vi "MasterSlaveDAQ-SplitMaster.vi"() -> ()   [LabVIEW 2014]
doc: "Use this template to build a user interface event handler design pattern. Use this pattern for dialog boxes and other user interfaces. You also can create and execute user-defined events that the VI can handle the same way as user interface events."
uses:
  subVIs/MasterState.ctl
  subVIs/SlaveStateData.ctl
  subVIs/SlaveState.ctl
  <vilib>/Utility/error.llb/DialogType.ctl
  <vilib>/DAQmx/create/channels.llb/DAQmx Create Channel (AI-Voltage-Basic).vi
  <vilib>/DAQmx/configure/timing.llb/DAQmx Timing (Sample Clock).vi
panel:
  in  "File Path":path
  in  "Acquire Data":bool
  in  "Log Data":bool
  in  "File Comment":string
  in  "DAQ Parameters":T1={"physical channels"="", "maximum value"=5.0, "minimum value"=-5.0, "rate"=1000.0, "read period"=0.5} {"read period" format="%0.2f"; "rate" format="%0.2f"; "minimum value" format="%0.2f"; "maximum value" format="%0.2f"}
  in  "quit":bool
  # "V"
  # "V"
  # "Hz"
  # "s"
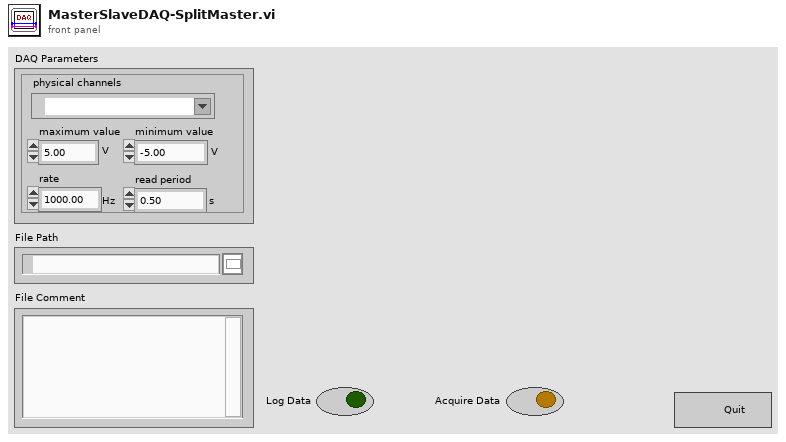
[diagram p1: front panel]
types:
  T1 = cluster{"physical channels":tag, "maximum value":dbl, "minimum value":dbl, "rate":dbl, "read period":dbl}
  T2 = typedef "SlaveStateData.ctl" = cluster{"New State":T3, "DAQ Ref":refnum<k21>, "File Ref":refnum<file>}
  T3 = typedef "SlaveState.ctl" = enum16{"Init", "Idle", "CheckError", "Finalize", "StartDAQ", "AcquireAndLog", "StopDAQ", "UpdateFile"}
  T4 = typedef "MasterState.ctl" = enum16{"Init", "Idle", "CheckError", "Finalize", "ConfigDAQ", "StartDAQ", "AcquireAndLog", "StopDAQ", "ClearDAQ", "OpenFile", "CloseFile"}
  T5 = typedef "DialogType.ctl" = u16
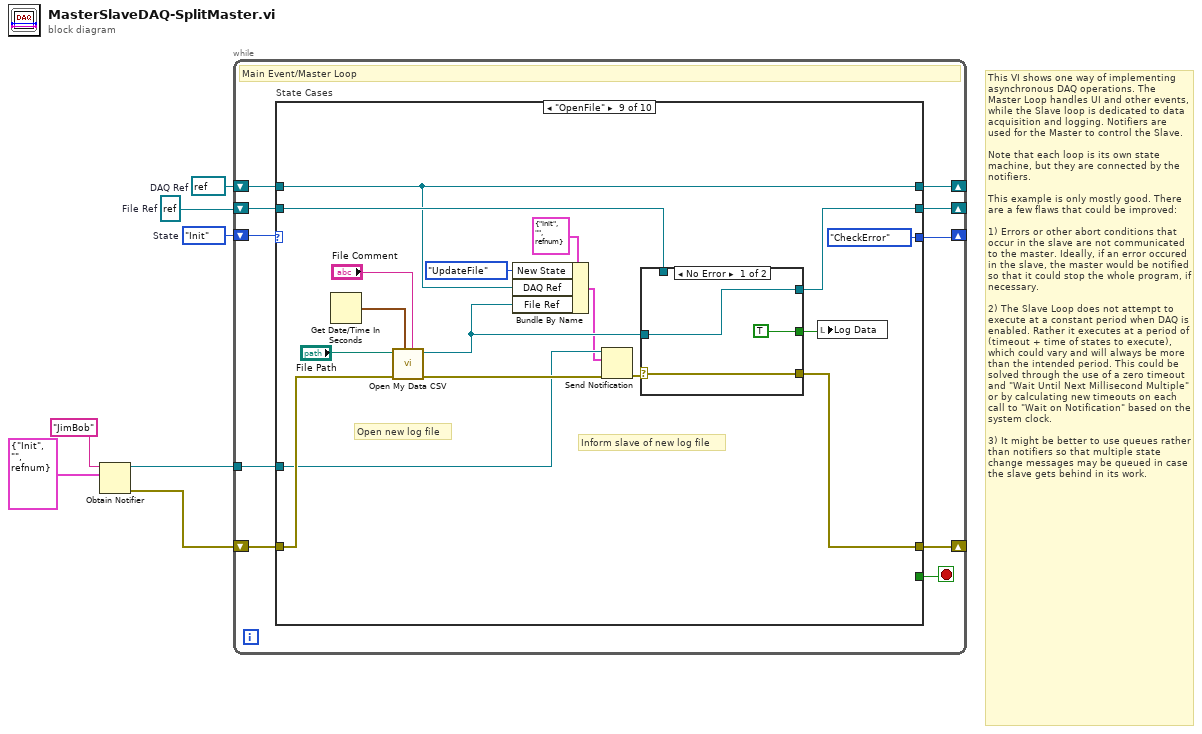
[diagram p0: block diagram]
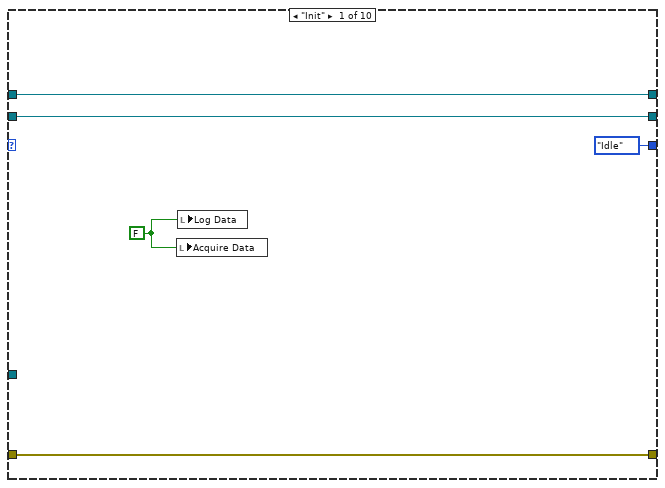
[diagram p2: hidden frame]
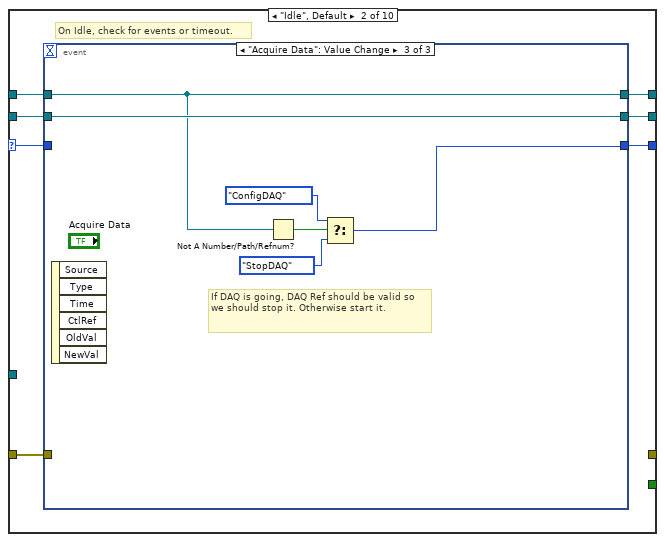
[diagram p3: hidden frame]
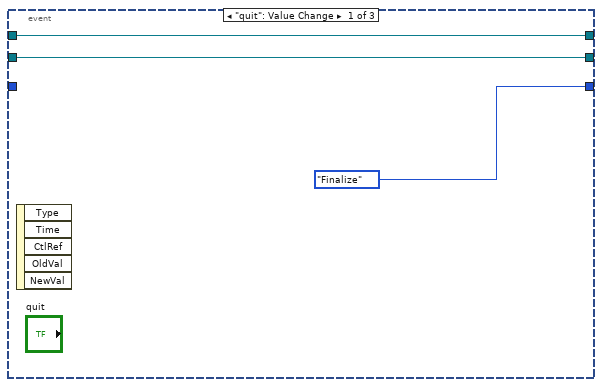
[diagram p4: hidden frame]
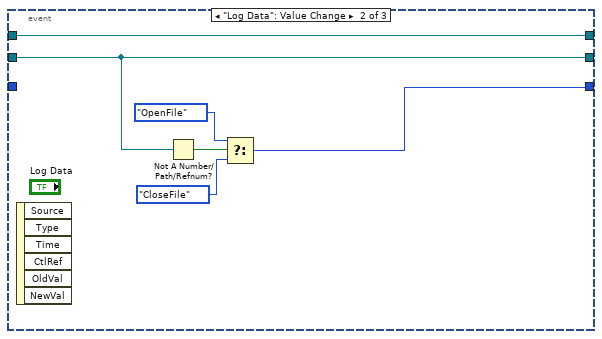
[diagram p5: hidden frame]
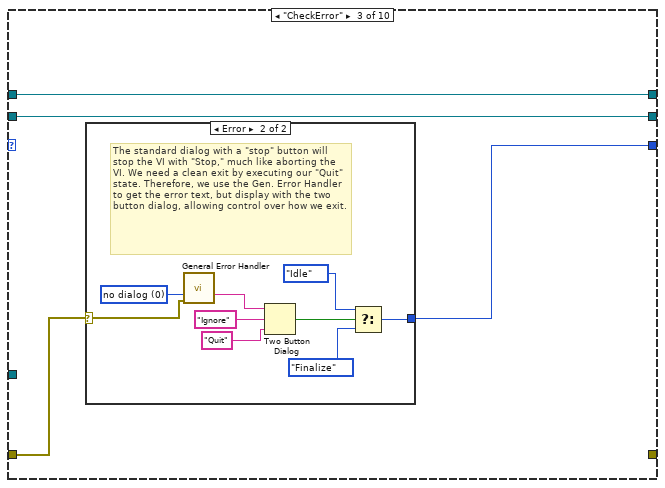
[diagram p6: hidden frame]
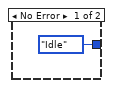
[diagram p7: hidden frame]
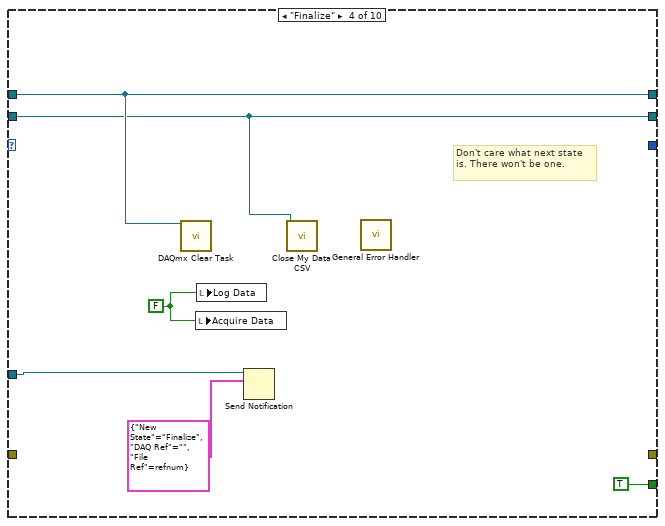
[diagram p8: hidden frame]
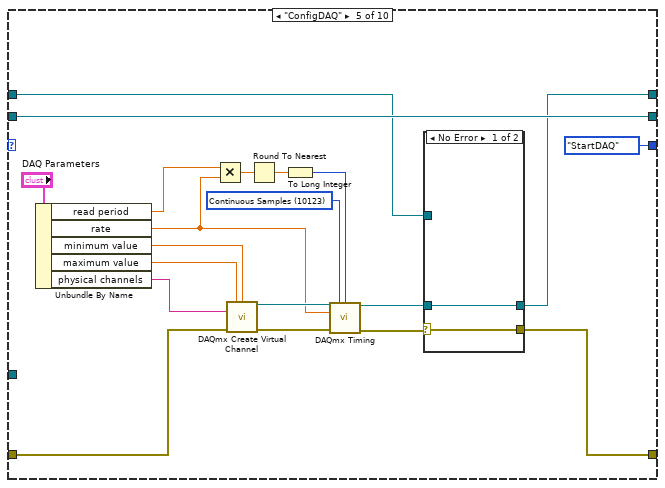
[diagram p9: hidden frame]
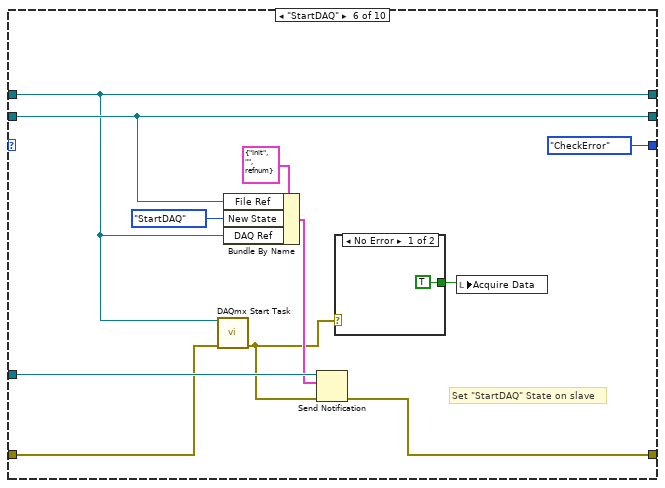
[diagram p11: hidden frame]
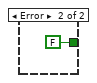
[diagram p12: hidden frame]
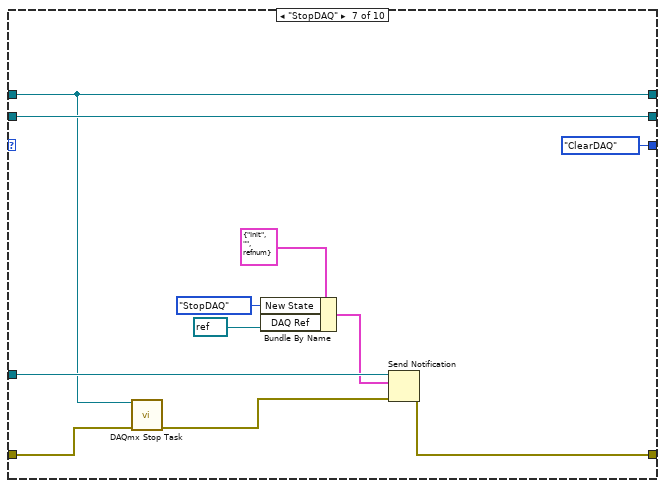
[diagram p13: hidden frame]
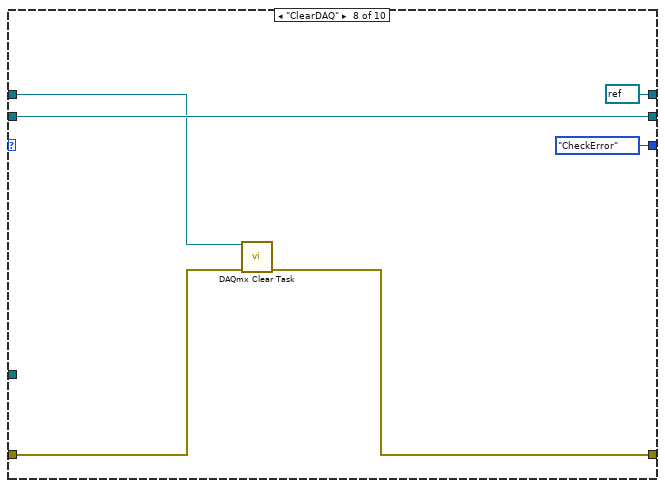
[diagram p14: hidden frame]
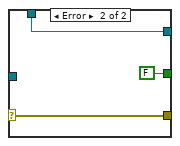
[diagram p15: hidden frame]
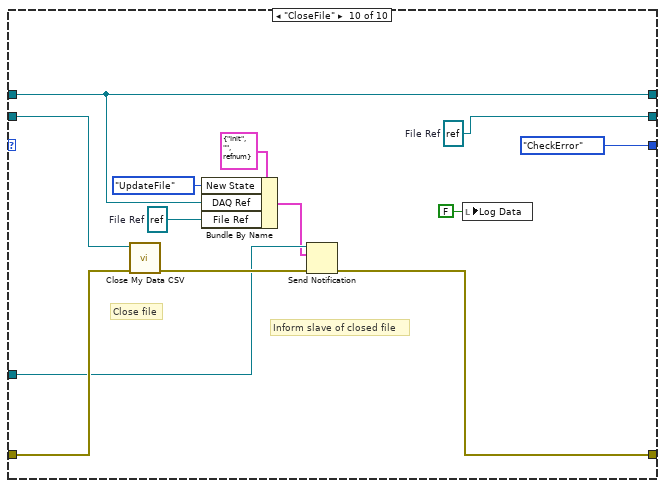
[diagram p16: hidden frame]
diagram:
  w5 = refnum<file> refnum  # File Ref
  w6 = refnum<k21> refnum  # DAQ Ref
  w7 = MasterState."Init"  # State
  # "This VI shows one way of implementing asynchronous DAQ operations. The Master Loop handles UI and other events, while the Slave loop is dedicated to data acquisition and logging. Notifiers are used for the Master to control the Slave.\n\nNote that each loop is its own state machine, but they are connected by the notifiers.\n\nThis example is only mostly good. There are a few flaws that could be improved:\n\n1) Errors or other abort conditions that occur in the slave are not communicated to the master. Ideally, if an error occured in the slave, the master would be notified so that it could stop the whole program, if necessary.\n\n2) The Slave Loop does not attempt to execute at a constant period when DAQ is enabled. Rather it executes at a period of (timeout + time of states to execute), which could vary and will always be more than the intended period. This could be solved through the use of a zero timeout and \"Wait Until Next Millisecond Multiple\" or by calculating new timeouts on each call to \"Wait on Notification\" based on the system clock.\n\n3) It might be better to use queues rather than notifiers so that multiple state change messages may be queued in case the slave gets behind in its work."
  n1 = Obtain Notifier(name (unnamed)="JimBob", notification data type=T2 {"New State"=enum."Init", "DAQ Ref"="", "File Ref"=refnum}) -> (notifier out=w4:refnum<notifier>, error out=w2:errorcluster)  [unwired: 2 in, 1 out]
  n2 = while {
    shift-right: [w16] -> _
    shift-left: w7 -> [w17]
    shift-right: [w15] -> _
    shift-left: w6 -> [w14]
    shift-right: [w13] -> _
    shift-left: w5 -> [w12]
    shift-right: [w11] -> _
    shift-left: w2 -> [w10]
    tunnel: w4 -> [w8]
    stop <- w9 stop-if-true
    # "Main Event/Master Loop"
    n3 = case "State Cases" shown="\"OpenFile\"" w17 {
      selector: w17 -> [_ w29 _ _ _ _ _ _ _ _]
      tunnel: [MasterState."Idle" ("State") w28 w46 _ MasterState."StartDAQ" ("State") MasterState."CheckError" ("State") MasterState."ClearDAQ" ("State") MasterState."CheckError" ("State") MasterState."CheckError" ("State") MasterState."CheckError" ("State")] -> w16
      tunnel: [w22 w25 w48 w63 w75 w91 w105 refnum<k21> refnum ("DAQ Ref") w121 w147] -> w15
      tunnel: w14 -> [w22 w24 w48 w63 w76 w91 w105 w115 w121 w147]
      tunnel: [w21 w27 w47 w62 w84 w94 w112 w117 w132 w151] -> w13
      tunnel: w12 -> [w21 w26 w47 w62 w84 w94 w112 w117 w122 w154]
      tunnel: [w18 _ _ _ w73 w95 w107 w113 w131 w144] -> w11
      tunnel: w10 -> [w18 w23 w45 _ w65 w92 w104 w114 w128 w150]
      tunnel: [_ _ _ TRUE _ _ _ _ _ _] -> w9
      tunnel: w8 -> [_ _ _ w60 _ w99 w111 _ w125 w143]
      frame "Init" {
        w19 = FALSE
        n4 = local write "Acquire Data"(w19) -> ()
        n5 = local write "Log Data"(w19) -> ()
      }
      frame "Idle", Default {
        # "On Idle, check for events or timeout."
        # "States"
        n6 = event shown="[2] \"Acquire Data\": Value Change" {
          selector: _ -> [_ _ _]
          dyn-events: _ -> [_ _ _]
          timeout: _ -> [_ _ _]
          tunnel: w29 -> [_ _ _]
          tunnel: [MasterState."Finalize" ("State") w33 w39] -> w28
          tunnel: [w31 w36 w44] -> w27
          tunnel: w26 -> [w31 w36 w44]
          tunnel: [w32 w38 w42] -> w25
          tunnel: w24 -> [w32 w38 w42]
          tunnel: w23 -> [_ _ _]
          event "quit": Value Change {
            n7 = event-data() -> ()  [unwired: 1 in, 5 out]
          }
          event "Log Data": Value Change {
            n8 = event-data() -> ()  [unwired: 1 in, 6 out]
            n9 = Not A Number/Path/Refnum?(number/path/refnum=w36) -> (NaN/Path/Refnum?=w37:bool)
            n10 = Select(t=MasterState."OpenFile" ("State"), s=w37, f=MasterState."CloseFile" ("State")) -> (s? t:f=w33:T4)
          }
          event "Acquire Data": Value Change {
            # "If DAQ is going, DAQ Ref should be valid so we should stop it. Otherwise start it."
            n11 = event-data() -> ()  [unwired: 1 in, 6 out]
            n12 = Not A Number/Path/Refnum?(number/path/refnum=w42) -> (NaN/Path/Refnum?=w43:bool)
            n13 = Select(t=MasterState."ConfigDAQ" ("State"), s=w43, f=MasterState."StopDAQ" ("State")) -> (s? t:f=w39:T4)
          }
        }
      }
      frame "CheckError" {
        n14 = case shown="Error" w45 {
          selector: w45 -> [_ w50]
          tunnel: [MasterState."Idle" ("State") w51] -> w46
          frame No Error {
          }
          frame Error {
            w58 = T5 0 items=["no dialog", "OK message", "continue or stop message", "OK message + warnings", "continue/stop + warnings"] ("type of dialog (OK msg:1)")
            # "The standard dialog with a \"stop\" button will stop the VI with \"Stop,\" much like aborting the VI. We need a clean exit by executing our \"Quit\" state. Therefore, we use the Gen. Error Handler to get the error text, but display with the two button dialog, allowing control over how we exit."
            n15 = call <vilib>:"General Error Handler.vi"("type of dialog (OK msg:1)"=w58, "error in (no error)"=w50) -> ("message"=w57:string)  [unwired: 9 in, 4 out]
            n16 = Two Button Dialog(message=w57, 1:"Quit" ("F button name (\"Cancel\")"), 2:"Ignore" ("T button name (\"OK\")")) -> (T button?=w54:bool)
            n17 = Select(t=MasterState."Idle" ("State"), s=w54, f=MasterState."Finalize" ("State")) -> (s? t:f=w51:T4)
          }
        }
      }
      frame "Finalize" {
        w61 = FALSE
        # "Don't care what next state is. There won't be one."
        n18 = call <vilib>:"DAQmx Clear Task.vi"("task in"=w63) -> ()  [unwired: 14 in, 1 out]
        n19 = local write "Acquire Data"(w61) -> ()
        n20 = local write "Log Data"(w61) -> ()
        n21 = Send Notification(notification=T2 {"New State"=enum."Finalize", "DAQ Ref"="", "File Ref"=refnum}, notifier=w60) -> ()  [unwired: 1 in, 2 out]
        n22 = call "Close My Data CSV.vi"("file refnum"=w62) -> ()  [unwired: 10 in, 1 out]
        n23 = call <vilib>:"General Error Handler.vi"() -> ()  [unwired: 11 in, 5 out]
      }
      frame "ConfigDAQ" {
        w81 = 10123 items=["Finite Samples"=10178, "Continuous Samples"=10123, "Hardware Timed Single Point"=12522] ("sample mode")
        n24 = Unbundle By Name("DAQ Parameters") -> ("read period"=w70:dbl, "rate"=w69:dbl, "minimum value"=w68:dbl, "maximum value"=w67:dbl, "physical channels"=w66:tag)
        n25 = Multiply(x=w70, y=w69) -> (x*y=w80:dbl)
        n26 = call-poly <vilib>:"DAQmx Create Virtual Channel.vi"("maximum value"=w67, "minimum value"=w68, "physical channels"=w66, "error in"=w65) -> ("task out"=w83:refnum<k21>, "error out"=w82:errorcluster)  [unwired: 10 in]
        n27 = Round To Nearest(number=w80) -> (nearest integer value=w79:dbl)
        n28 = To Long Integer(number=w79) -> (32bit integer=w78:i32)
        n29 = call-poly <vilib>:"DAQmx Timing.vi"("task/channels in"=w83, "sample mode"=w81, "samples per channel"=w78, "rate"=w69, "error in"=w82) -> ("task out"=w74:refnum<k21>, "error out"=w77:errorcluster)  [unwired: 9 in]
        n30 = case shown="No Error" w77 {
          selector: w77 -> [w85 w88]
          tunnel: w76 -> [_ w87]
          tunnel: [w86 w87] -> w75
          tunnel: w74 -> [w86 _]
          tunnel: [w85 w88] -> w73
          frame No Error {
          }
          frame Error {
          }
        }
      }
      frame "StartDAQ" {
        # "Set \"StartDAQ\" State on slave"
        n31 = call <vilib>:"DAQmx Start Task.vi"("task/channels in"=w91, "error in"=w92) -> ("error out"=w90:errorcluster)  [unwired: 12 in, 1 out]
        n32 = Bundle By Name(cluster=T2 {"New State"=enum."Init", "DAQ Ref"="", "File Ref"=refnum} ("notification"), "File Ref"=w94, "New State"=SlaveState."StartDAQ", "DAQ Ref"=w91) -> (w96:T2)
        n33 = Send Notification(notification=w96, notifier=w99, error in (no error)=w90) -> (error out=w95:errorcluster)  [unwired: 1 out]
        n34 = case shown="No Error" w90 {
          tunnel: [TRUE FALSE] -> w89
          frame No Error {
          }
          frame Error {
          }
        }
        n35 = local write "Acquire Data"(w89) -> ()
      }
      frame "StopDAQ" {
        n36 = call <vilib>:"DAQmx Stop Task.vi"("task/channels in"=w105, "error in"=w104) -> ("error out"=w103:errorcluster)  [unwired: 12 in, 1 out]
        n37 = Bundle By Name(cluster=T2 {"New State"=enum."Init", "DAQ Ref"="", "File Ref"=refnum} ("notification"), "New State"=SlaveState."StopDAQ", "DAQ Ref"=refnum<k21> refnum) -> (w108:T2)
        n38 = Send Notification(notification=w108, notifier=w111, error in (no error)=w103) -> (error out=w107:errorcluster)  [unwired: 1 out]
      }
      frame "ClearDAQ" {
        n39 = call <vilib>:"DAQmx Clear Task.vi"("task in"=w115, "error in"=w114) -> ("error out"=w113:errorcluster)  [unwired: 13 in]
      }
      frame "OpenFile" {
        # "Open new log file"
        # "Inform slave of new log file"
        n40 = Get Date/Time In Seconds() -> (seconds since 1Jan1904=w135:timestamp)
        n41 = call "Open My Data CSV.vi"("Comment"="File Comment", "Time Stamp"=w135, "error in"=w128, "file path"="File Path") -> ("error out"=w127:errorcluster, "refnum out"=w120:refnum<file>)  [unwired: 6 in]
        n42 = Bundle By Name(cluster=T2 {"New State"=enum."Init", "DAQ Ref"="", "File Ref"=refnum} ("notification"), "New State"=SlaveState."UpdateFile", "DAQ Ref"=w121, "File Ref"=w120) -> (w119:T2)
        n43 = Send Notification(notification=w119, notifier=w125, error in (no error)=w127) -> (error out=w126:errorcluster)  [unwired: 1 out]
        n44 = case shown="No Error" w126 {
          selector: w126 -> [w137 w141]
          tunnel: [w138 w139] -> w132
          tunnel: w120 -> [w138 _]
          tunnel: [w137 w141] -> w131
          tunnel: [TRUE ("Log Data") FALSE ("Log Data")] -> w130
          tunnel: w122 -> [_ w139]
          frame No Error {
          }
          frame Error {
          }
        }
        n45 = local write "Log Data"(w130) -> ()
      }
      frame "CloseFile" {
        w146 = refnum<file> refnum  # File Ref
        w151 = refnum<file> refnum  # File Ref
        # "Close file"
        # "Inform slave of closed file"
        n46 = call "Close My Data CSV.vi"("error in"=w150, "file refnum"=w154) -> ("error out"=w145:errorcluster)  [unwired: 9 in]
        n47 = Bundle By Name(cluster=T2 {"New State"=enum."Init", "DAQ Ref"="", "File Ref"=refnum} ("notification"), "New State"=SlaveState."UpdateFile", "DAQ Ref"=w147, "File Ref"=w146) -> (w142:T2)
        n48 = Send Notification(notification=w142, notifier=w143, error in (no error)=w145) -> (error out=w144:errorcluster)  [unwired: 1 out]
        n49 = local write "Log Data"(FALSE ("Log Data")) -> ()
      }
    }
  }
